vi "Stop Core.vi"(10 "final error code":i32, 11 "Nested in":refnum<class "FC2901.lvclass">) -> (3 "Nested out":refnum<class "FC2901.lvclass">)   [LabVIEW 2021, in "FC2901.lvclass"]
doc: "(<B>Filename</B>: Actor Framework.lvlib:Actor.lvclass:Stop Core.vi)\n\nDefines what the actor does before it stops. Use the <B>final error code</B> input to determine whether the actor shut down in response to an error.\n\nBy default, this method does nothing. A descendant class may override it to define behavior, such as shutting down any processes the actor initiated in its override of the Actor Core method."
uses:
  FC2901.lvclass
  <vilib>/MGI/Panel Manager/Panel Actor/Panel Actor/Panel Actor.lvclass
  FC2901.lvclass/FC2901.ctl
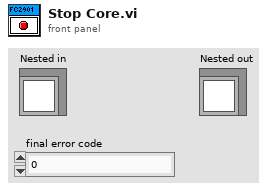
[diagram p1: front panel]
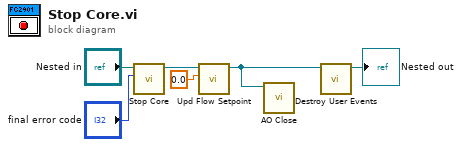
[diagram p0: block diagram]
diagram:
  n1 = call-parent "Stop Core.vi"("final error code"="final error code", "Actor in"="Nested in") -> ("Actor out"=w3:refnum<class "FC2901.lvclass">)  [unwired: 9 in]
  n2 = call "Upd Flow Setpoint.vi"("Flow Setpoint"=0.0, "C100L in"=w3) -> ("C100L out"=w1:refnum<class "FC2901.lvclass">)  [unwired: 8 in, 1 out]
  n3 = call "AO Close.vi"("C100L in"=w1) -> ()  [unwired: 10 in, 1 out]
  n4 = call "Destroy User Events.vi"("UI Template in"=w1) -> ("UI Template out"=→"Nested out":refnum<class "FC2901.lvclass">)  [unwired: 10 in]
